vi "Parse Data.vi"(11 "Data In":u64[](array[numeric])) -> (2 "Values to Log":string[][](array[string]), 3 "Histogram Data":i16[](array[numeric]))   [LabVIEW 2017]
panel:
  out "Array":i16[][](array[numeric])
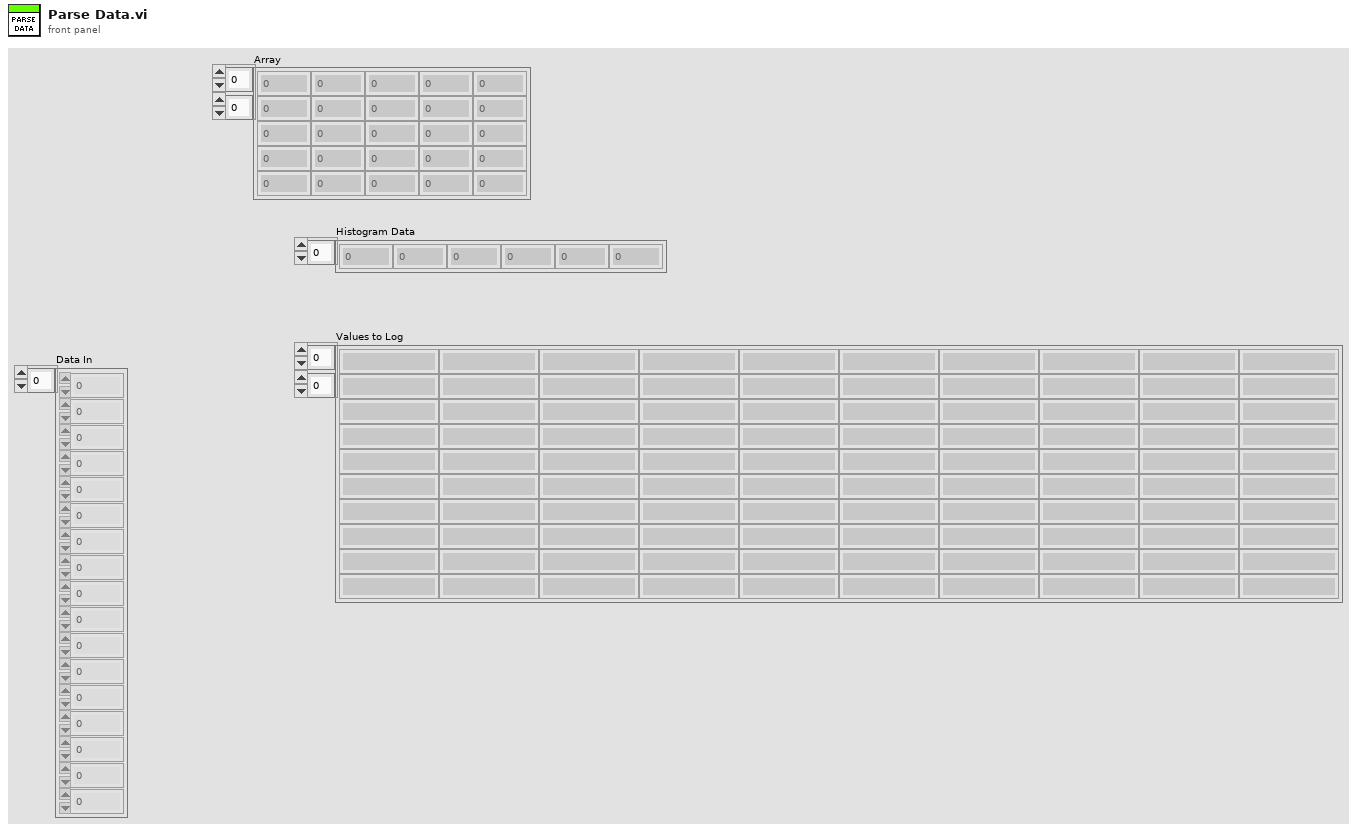
[diagram p1: front panel]
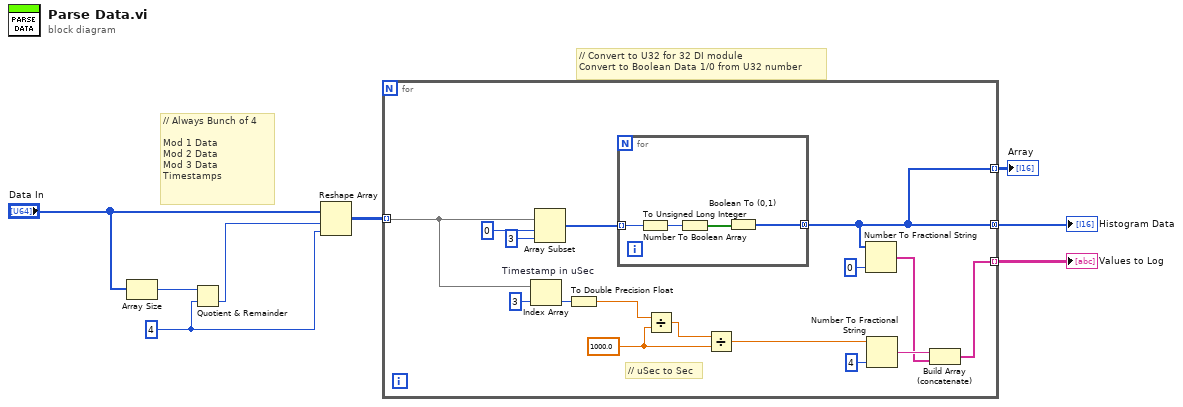
[diagram p0: block diagram]
diagram:
  w7 = 4 ("y")
  # "// Convert to U32 for 32 DI module\nConvert to Boolean Data 1/0 from U32 number"
  # "// Always Bunch of 4\n\nMod 1 Data\nMod 2 Data\nMod 3 Data\nTimestamps"
  n1 = Array Size(array="Data In") -> (size(s)=w4:i32)
  n2 = Quotient & Remainder(x=w4, y=w7) -> (floor(x/y)=w6:i32)  [unwired: 1 out]
  n3 = Reshape Array("Data In", w6, w7) -> (w8:u64[][])
  n4 = for {
    tunnel: w8 -> [w22] mode=indexing
    tunnel: [w9] -> w2 mode=concatenating
    tunnel: [w12] -> w3 mode=indexing
    tunnel: [w9] -> w1 mode=indexing
    w17 = 1000.0 ("y")
    # "// uSec to Sec"
    n5 = Index Array "Timestamp in uSec"(array=w22, index=3) -> (element=w20:u64)
    n6 = Array Subset(array=w22, index=0, length=3) -> (w16:u64[])
    n7 = To Double Precision Float(number=w20) -> (double precision float=w19:dbl)
    n8 = for {
      tunnel: w16 -> [w27] mode=indexing
      tunnel: [w25] -> w9 mode=concatenating
      n9 = To Unsigned Long Integer(number=w27) -> (unsigned 32bit integer=w26:u32)
      n10 = Number To Boolean Array(number=w26) -> (Boolean array=w28:bool[])
      n11 = Boolean To (0,1)(Boolean=w28) -> (0, 1=w25:i16[])
    }
    n12 = Divide(x=w19, y=w17) -> (x/y=w18:dbl)
    n13 = Divide(x=w18, y=w17) -> (x/y=w13:dbl)
    n14 = Number To Fractional String(number=w9, precision (6)=i16 0) -> (F-format string=w10:string[])  [unwired: 2 in]
    n15 = Number To Fractional String(number=w13, precision (6)=i16 4) -> (F-format string=w11:string)  [unwired: 2 in]
    n16 = Build Array (concatenate)(w11, w10) -> (w12:string[])
  }
  "Values to Log" <- w3
  "Histogram Data" <- w2
  "Array" <- w1
